vi "CrossProduct.vi"(1 "V2":dbl[](array[numeric]), 2 "V1":dbl[](array[numeric])) -> (0 "V1^V2":dbl[](array[numeric]))   [LabVIEW 2009]
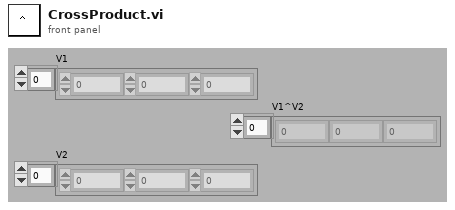
[diagram p1: front panel]
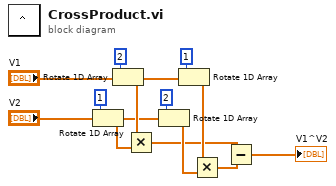
[diagram p0: block diagram]
diagram:
  n1 = Rotate 1D Array(1:"V2", 2:1 ("n")) -> (0:w10:dbl[])
  n2 = Rotate 1D Array(1:"V1", 2:2 ("n")) -> (0:w11:dbl[])
  n3 = Multiply(x=w11, y=w10) -> (x*y=w3:dbl[])
  n4 = Rotate 1D Array(1:"V2", 2:2 ("n")) -> (0:w9:dbl[])
  n5 = Rotate 1D Array(1:"V1", 2:1 ("n")) -> (0:w8:dbl[])
  n6 = Multiply(x=w8, y=w9) -> (x*y=w2:dbl[])
  n7 = Subtract(x=w3, y=w2) -> (x-y=→"V1^V2":dbl[])
